vi "CHECK_Condition_has_been_set.vi"(2 "error in (no error)":T1, 3 "Current condition cluster in":T2 caption="Condition" {"Specifier(s)"."Validity criteria(s)"."Validity value" min=0.0 step=0.1 format="%.2g"; "Specifier(s)"."Value" step=1.0 format="%#.2g"}) -> (0 "error out":T1, 1 "Has been set before?":bool)   [LabVIEW 2018, in "Tracker.lvlib"]
uses:
  Tracker.lvlib
  Controls/CTL_Conditions_Cluster.ctl
  Controls/CTL_Condition_type.ctl
  Controls/CTL_Comparison_type.ctl
  Controls/CTL_Validity_check_criteria.ctl
  Controls/CTL_Response_info.ctl
  Controls/CTL_Condition_response_type.ctl
  Controls/CTL_Reponse_port_info.ctl
  Common_Resources.lvlib
panel:
  out "element":T2 caption="Condition" {"Specifier(s)"."Validity criteria(s)"."Validity value" min=0.0 step=0.1 format="%.2g"; "Specifier(s)"."Value" step=1.0 format="%#.2g"}
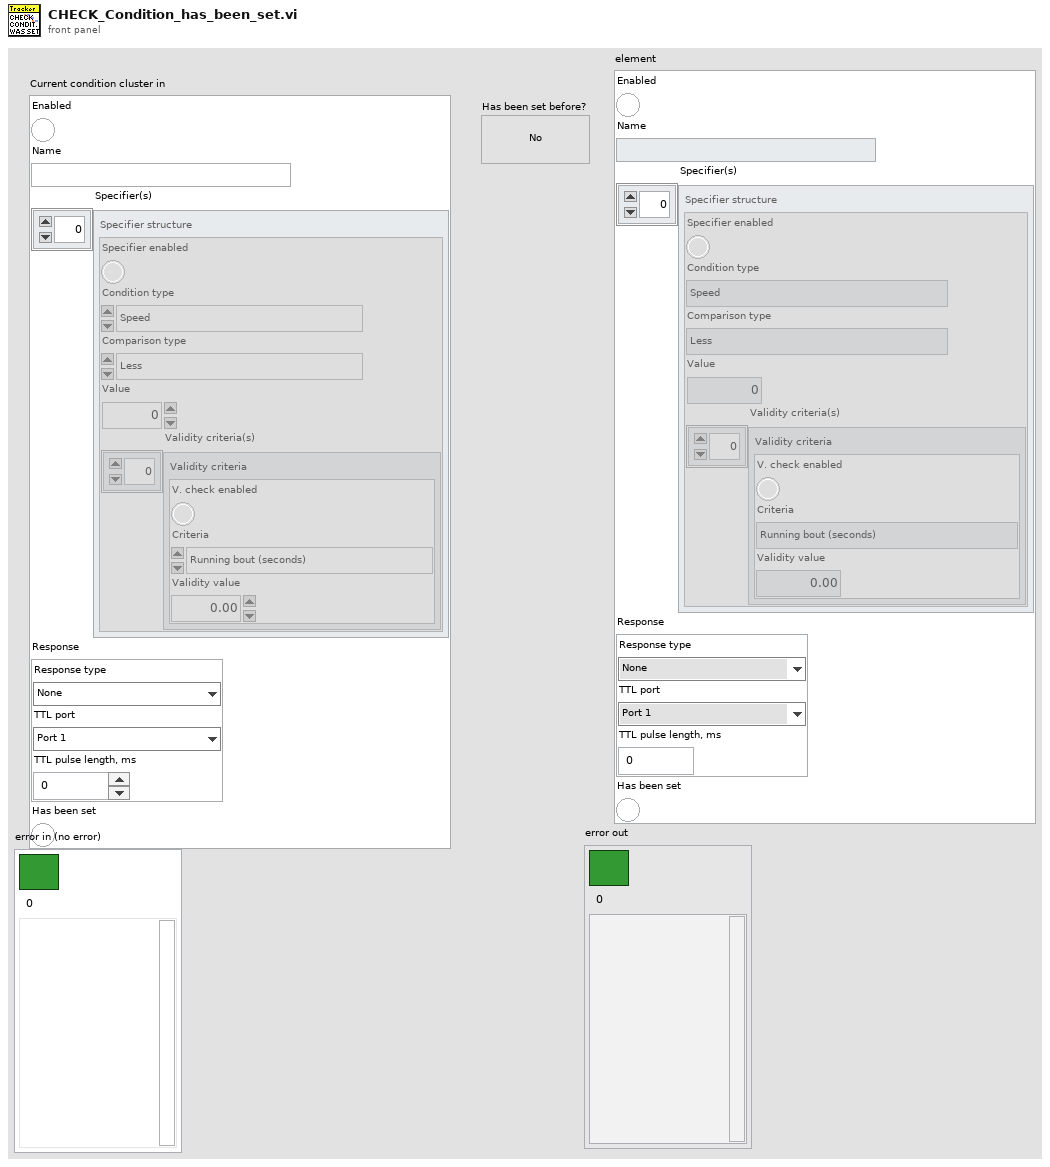
[diagram p1: front panel]
types:
  T1 = cluster{"Boolean Round":bool, "code":i32, "source":string}
  T2 = typedef "Common_Resources.lvlib/CTL_Conditions_Cluster.ctl" = cluster{"Enabled":bool, "Name":string, "Specifier(s)":cluster{"Specifier enabled":bool, "Condition type":T3, "Comparison type":T4, "Value":dbl, "Validity criteria(s)":cluster{"V. check enabled":bool, "Criteria":T5, "Validity value":dbl}[]}[], "Response":T6, "Has been set":bool}
  T3 = typedef "Common_Resources.lvlib/CTL_Condition_type.ctl" = enum16{"Speed", "Zone", "Angle to wall"}
  T4 = typedef "Common_Resources.lvlib/CTL_Comparison_type.ctl" = enum16{"Less", "Less or Equal", "Equal", "Greater or Equal", "Greater", "Not Equal"}
  T5 = typedef "Common_Resources.lvlib/CTL_Validity_check_criteria.ctl" = enum16{"Running bout (seconds)", "Running bout (meters)"}
  T6 = typedef "Common_Resources.lvlib/CTL_Response_info.ctl" = cluster{"Response type":T7, "TTL port":T8, "TTL pulse length, ms":dbl}
  T7 = typedef "Common_Resources.lvlib/CTL_Condition_response_type.ctl" = enum16{"None", "Air puff", "Liquid reward"}
  T8 = typedef "Common_Resources.lvlib/CTL_Reponse_port_info.ctl" = enum16{"Port 1", "Port 2", "Port 3", "Port 4"}
  T9 = typedef "Common_Resources.lvlib/CTL_Conditions_Array.ctl" = T2[]
  T10 = cluster{"Specifier enabled":bool, "Condition type":T3, "Comparison type":T4, "Value":dbl, "Validity criteria(s)":cluster{"V. check enabled":bool, "Criteria":T5, "Validity value":dbl}[]}[]
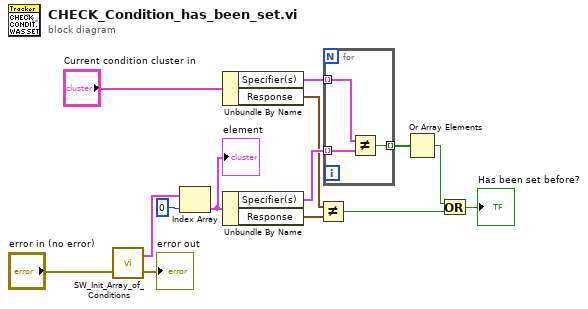
[diagram p0: block diagram]
diagram:
  n1 = call "SW_Init_Array_of_Conditions.vi"("error in (no error)"="error in (no error)") -> ("error out"=→"error out":T1, "Array of conditions"=w7:T9)  [unwired: 1 in]
  n2 = Index Array(array=w7, index=0) -> (element=w5:T2)
  "element" <- w5
  n3 = Unbundle By Name("Current condition cluster in") -> ("Specifier(s)"=w13:T10, "Response"=w11:T6)
  n4 = Unbundle By Name(w5) -> ("Specifier(s)"=w12:T10, "Response"=w10:T6)
  n5 = Not Equal?(x=w11, y=w10) -> (x != y?=w8:bool)
  n6 = for {
    tunnel: w13 -> [w17] mode=indexing
    tunnel: w12 -> [w16] mode=indexing
    tunnel: [w15] -> w4 mode=indexing
    n7 = Not Equal?(x=w17, y=w16) -> (x != y?=w15:bool)
  }
  n8 = Or Array Elements(Boolean array=w4) -> (logical OR=w3:bool)
  n9 = Or(x=w3, y=w8) -> (x .or. y?=→"Has been set before?":bool)
